vi "Global_ACT Write_Data Out.vi"() -> ()   [LabVIEW 2017, in "Arm.lvlib"]
uses:
  Arm.lvlib
  CLUSTER_ElbowOutput.ctl
panel:
  out "Arm_ACT_Wrist_Output":T1
  out "Arm_ACT_Telescope_Output":T1
  out "Arm_ACT_Elbow_Output":T1
  # "The Names of the Data items in the Global Variable MUST describe who the Single Writer is\nNaming Convention of all Data Items is:   \nLib Name_Loop Name (SM or SEN or ACT)_Data Name\nExamples:\nDrive_ACT_X axis\nGameController_SEN_JoystickLeft\nHopper_SM_AgitatorSpeed"
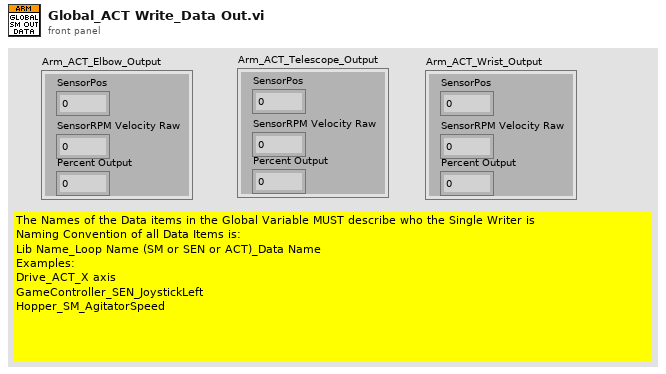
[diagram p1: front panel]
types:
  T1 = typedef "Arm.lvlib/CLUSTER_ElbowOutput.ctl" = cluster{"SensorPos":i32, "SensorRPM Velocity Raw":i32, "Percent Output":dbl}
diagram:
